vi "Write.vi"(4 "Full Scale Voltage (4.096)":dbl=4.096, 6 "DAC Resolution Ticks (4096)":dbl=4096.0, 7 "I2C Channel":u8, 8 "Error In":errorcluster, 9 "Voltage (V)":dbl, 10 "I2C Slave Address (0)":u8, 11 "LINX Resource":T1={"IO"=enum."Remote", "Interface"=enum."TCP", "LINX Device Config"={"Interface"=enum."TCP", "COM Port"="N/A", "TCP Configuration"={"IP Address"="panicattack", "Port"=6999}, "Device Family"=4, "Device ID"=1, "Device Name"="Raspberry Pi Model B", "TCP Ref"=refnum, "Channels"={"DI"=[2, 3, 4, 7, 8, 9, 10, 11, 14, 15, 17, 18, 22, 23, 24, 25, 27], "DO"=[2, 3, 4, 7, 8, 9, 10, 11, 14, 15, 17, 18, 22, 23, 24, 25, 27], "AI"=[], "AO"=[], "PWM"=[], "QE"=[], "UART"=[0], "I2C 2"=[0, 1], "SPI"=[0], "CAN"=[], "Servo"=[], "AI Ref (V)"=0.0, "AI Resolution (Bits)"=0, "AO Ref (V)"=0.0, "AO Resolution (Bits)"=0}}}) -> (0 "Error Out":errorcluster, 3 "LINX Resource":T1={"IO"=enum."Remote", "Interface"=enum."TCP", "LINX Device Config"={"Interface"=enum."TCP", "COM Port"="N/A", "TCP Configuration"={"IP Address"="panicattack", "Port"=6999}, "Device Family"=4, "Device ID"=1, "Device Name"="Raspberry Pi Model B", "TCP Ref"=refnum, "Channels"={"DI"=[2, 3, 4, 7, 8, 9, 10, 11, 14, 15, 17, 18, 22, 23, 24, 25, 27], "DO"=[2, 3, 4, 7, 8, 9, 10, 11, 14, 15, 17, 18, 22, 23, 24, 25, 27], "AI"=[], "AO"=[], "PWM"=[], "QE"=[], "UART"=[0], "I2C 2"=[0, 1], "SPI"=[0], "CAN"=[], "Servo"=[], "AI Ref (V)"=0.0, "AI Resolution (Bits)"=0, "AO Ref (V)"=0.0, "AO Resolution (Bits)"=0}}})   [LabVIEW 2020, in "LMH-LINX.lvlib" / "LTC2631.lvlib"]
doc: "Write the specified output voltage to the LTC2631. \n\nDAC Resolution Ticks is used to set the number of DAC ticks and should be equal to 2^Resolution. The default is 4096 (12-bit)\n\nFull Scale Voltage is the full scale voltage range the the DAC is capable of outputtting. This depends on the DAC model and supply voltage."
uses:
  LTC2631.lvlib
  Private/Type Defs/LINX Ref.ctl
  Private/Type Defs/Platform.ctl
  Private/Type Defs/Interface.ctl
  Private/Device/Type Defs/LINX Device Config.ctl
  Private/Device/Type Defs/TCP Config.ctl
  Private/Device/Type Defs/Channels.ctl
  Utilities/Check Channel.vi
  Private/Utilties/Generate Error.vi
  LMH-LINX.lvlib
  Private/Device/Device.lvlib
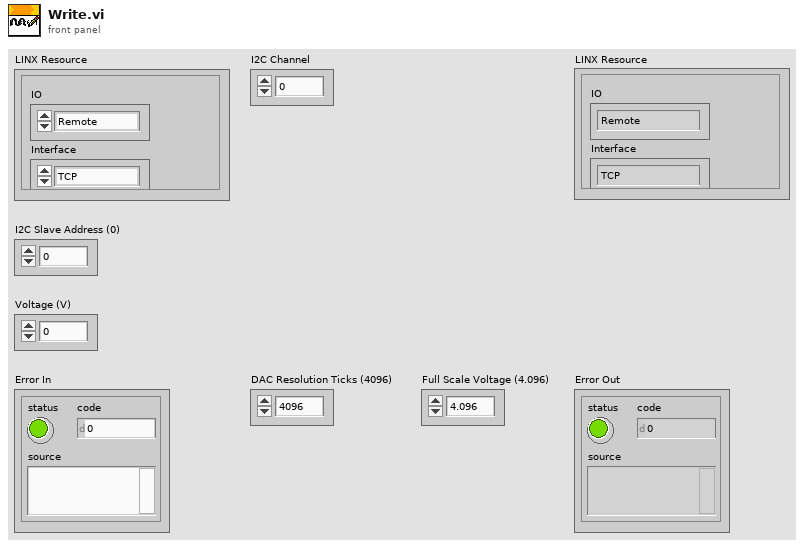
[diagram p1: front panel]
types:
  T1 = typedef "LMH-LINX.lvlib/LINX Ref.ctl" = cluster{"IO":T2, "Interface":T3, "LINX Device Config":T4}
  T2 = typedef "LMH-LINX.lvlib/Platform.ctl" = enum16{"Remote", "Local"}
  T3 = typedef "LMH-LINX.lvlib/Interface.ctl" = enum16{"Serial", "TCP"}
  T4 = typedef "Device.lvlib/LINX Device Config.ctl" = cluster{"Interface":T3, "COM Port":refnum<visa-resource-name>, "TCP Configuration":T5, "Device Family":u8, "Device ID":u8, "Device Name":string, "TCP Ref":refnum<k5>, "Channels":T6}
  T5 = typedef "Device.lvlib/TCP Config.ctl" = cluster{"IP Address":string, "Port":u16}
  T6 = typedef "LMH-LINX.lvlib/Channels.ctl" = cluster{"DI":u8[], "DO":u8[], "AI":u8[], "AO":u8[], "PWM":u8[], "QE":u8[], "UART":u8[], "I2C 2":u8[], "SPI":u8[], "CAN":u8[], "Servo":u8[], "AI Ref (V)":dbl, "AI Resolution (Bits)":u8, "AO Ref (V)":dbl, "AO Resolution (Bits)":u8}
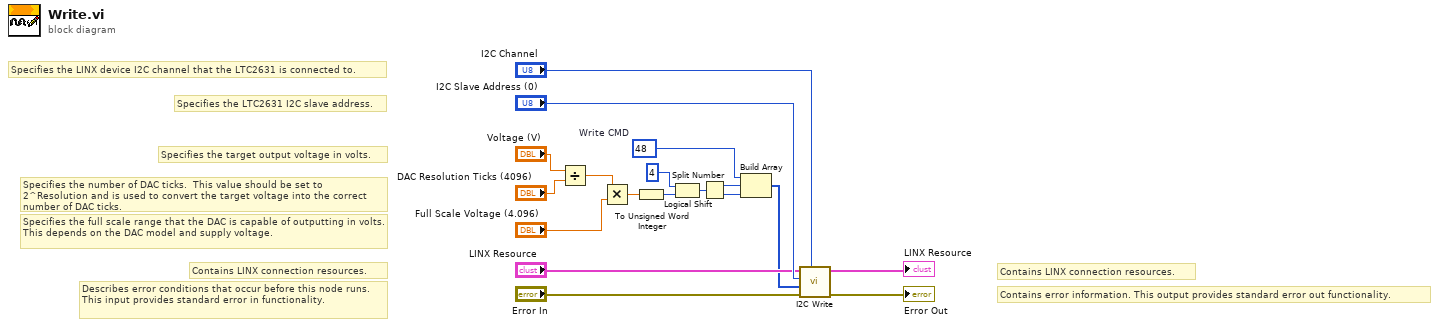
[diagram p0: block diagram]
diagram:
  w2 = u8 48  # Write CMD
  # "Specifies the LTC2631 I2C slave address."
  # "Specifies the LINX device I2C channel that the LTC2631 is connected to."
  # "Specifies the target output voltage in volts."
  # "Specifies the number of DAC ticks.  This value should be set to 2^Resolution and is used to convert the target voltage into the correct number of DAC ticks."
  # "Specifies the full scale range that the DAC is capable of outputting in volts. This depends on the DAC model and supply voltage."
  # "Contains LINX connection resources."
  # "Contains error information. This output provides standard error out functionality."
  # "Contains LINX connection resources."
  # "Describes error conditions that occur before this node runs. This input provides standard error in functionality."
  n1 = Divide(x="Voltage (V)", y="DAC Resolution Ticks (4096)") -> (x/y=w10:dbl)
  n2 = Multiply(x=w10, y="Full Scale Voltage (4.096)") -> (x*y=w8:dbl)
  n3 = To Unsigned Word Integer(number=w8) -> (unsigned 16bit integer=w7:u16)
  n4 = Logical Shift(y=i8 4, x=w7) -> (x << y=w5:u16)
  n5 = Split Number(x=w5) -> (hi(x)=w4:u8, lo(x)=w3:u8)
  n6 = Build Array(w2, w4, w3) -> (w1:u8[])
  n7 = call "I2C Write.vi"("I2C Channel"="I2C Channel", "Error In"="Error In", "Data"=w1, "I2C Slave Address (0)"="I2C Slave Address (0)", "LINX Resource"="LINX Resource") -> ("Error Out"=→"Error Out":errorcluster, "LINX Resource"=→"LINX Resource":T1)  [unwired: 5 in]
